vi "Callback - Get Data by Name.vi"(8 "error in (no error)":errorcluster, 9 "Oldest Time to Plot":dbl, 10 "Name":string, 11 "BluePlotHandleDemo in":refnum<class "BluePlotHandleDemo.lvclass">) -> (0 "error out":errorcluster, 2 "data history":T1, 3 "BluePlotHandleDemo out":refnum<class "BluePlotHandleDemo.lvclass">)   [LabVIEW 2021, in "BluePlotDemo.lvlib" / "BluePlotHandleDemo.lvclass"]
uses:
  BluePlotHandleDemo.lvclass
  TypeDefs/plot datapoint.ctl
  SubVIs/Demo Names.ctl
  BluePlotHandleDemo.lvclass/BluePlotHandleDemo.ctl
  SubVIs/ring buffer data.ctl
  BluePlotDemo.lvlib
  <vilib>/National Instruments/Variant Ring Buffer/Ring Buffer.lvclass
  BluePlot.lvlib
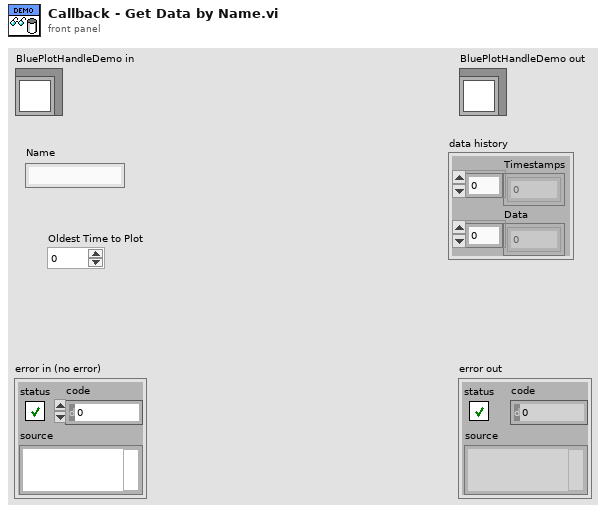
[diagram p1: front panel]
types:
  T1 = typedef "BluePlot.lvlib/plot datapoint.ctl" = cluster{"Timestamps":dbl[], "Data":dbl[]}
  T2 = typedef "BluePlotDemo.lvlib/Demo Names.ctl" = enum16{"Sine Wave", "Triangle Wave", "Sawtooth Wave", "Square Wave", "Uniform Noise", "Periodic Noise", "White Noise"}
  T3 = typedef "BluePlotDemo.lvlib/ring buffer data.ctl" = cluster{"timestamp":dbl, "value":dbl}
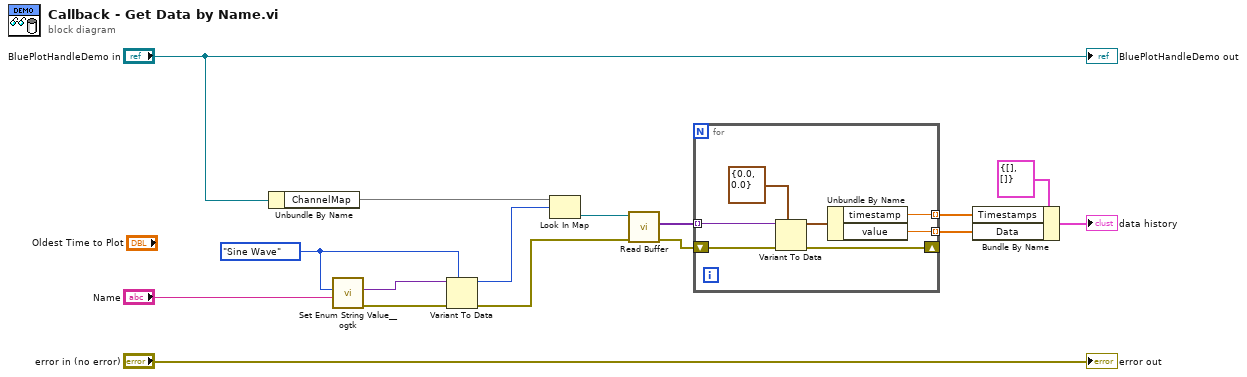
[diagram p0: block diagram]
diagram:
  w13 = Demo_Names."Sine Wave" ("channel")
  n1 = Unbundle By Name("BluePlotHandleDemo in") -> ("ChannelMap"=w11:map{T2, refnum<data-value>})
  n2 = call <userlib>:"Set Enum String Value__ogtk.vi"("String Value"="Name", "Default Enum Value"=w13) -> ("error out"=w14:errorcluster, "Enum"=w15:variant)  [unwired: 8 in]
  n3 = Variant To Data(error in=w14, type=w13, Variant=w15) -> (data=w10:T2, error out=w3:errorcluster)
  n4 = Look In Map(map=w11, key=w10) -> (value=w9:refnum<data-value>)  [unwired: 1 in, 1 out]
  n5 = call <vilib>:"Read Buffer.vi"("Error In"=w3, "Ring Buffer Reference"=w9) -> ("Error Out"=w2:errorcluster, "Array of Variants"=w8:variant[])  [unwired: 7 in, 1 out]
  n6 = for {
    tunnel: w8 -> [w23] mode=indexing
    tunnel: [w20] -> w6 mode=indexing
    tunnel: [w19] -> w5 mode=indexing
    shift-right: [w17] -> _
    shift-left: w2 -> [w18]
    n7 = Variant To Data(error in=w18, type=T3 {"timestamp"=0.0, "value"=0.0} ("Cluster"), Variant=w23) -> (data=w21:T3, error out=w17:errorcluster)
    n8 = Unbundle By Name(w21) -> ("timestamp"=w20:dbl, "value"=w19:dbl)
  }
  n9 = Bundle By Name(cluster=T1 {"Timestamps"=[], "Data"=[]} ("data history"), "Timestamps"=w6, "Data"=w5) -> (→"data history":T1)
  "error out" <- "error in (no error)"
  "BluePlotHandleDemo out" <- "BluePlotHandleDemo in"
